vi "test_MultipleSessionsReserved_CallCreateSession_ReturnsErrorForTooManySessions.vi"(8 "error in":errorcluster) -> (0 "error out":errorcluster, 2 "result":string, 3 "pass":bool)   [LabVIEW 2020, in "MeasurementServerTests.lvlib"]
uses:
  MeasurementServerTests.lvlib
  3a947300-8ba6-4980-845e-9b7eeaceb0a3.vi
  Helpers/Fake Instrument/Fake Instrument.lvclass
  \\tsclient\C/dev/measurementlink-labview/Source/Runtime/MeasurementLink Instrument/IInstrument/IInstrument.lvclass
  Runtime/MeasurementLink Measurement Server/Helpers/Error Strings Global Internal.vi
  Runtime/MeasurementLink Session Management/Session Reservation/Create Sessions Impl.vi
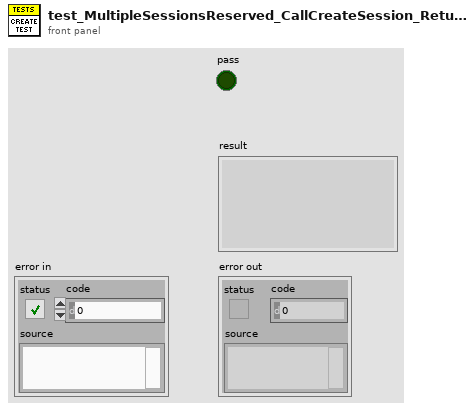
[diagram p1: front panel]
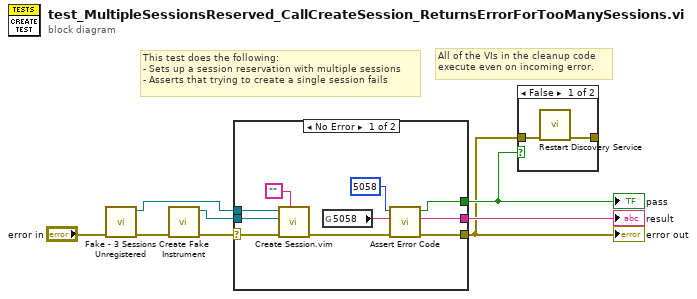
[diagram p0: block diagram]
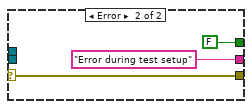
[diagram p2: hidden frame]
diagram:
  # "All of the VIs in the cleanup code\nexecute even on incoming error."
  # "This test does the following:\n- Sets up a session reservation with multiple sessions\n- Asserts that trying to create a single session fails"
  n1 = call "Fake - 3 Sessions Unregistered.vi"("error in"="error in") -> ("error out"=w2:errorcluster, "session reservation out"=w1:refnum<class "Session Reservation.lvclass">)  [unwired: 9 in]
  n2 = call "Create Fake Instrument.vi"("error in"=w2) -> ("error out"=w5:errorcluster, "fake instrument out"=w4:refnum<class "Fake Instrument.lvclass">)  [unwired: 9 in]
  n3 = case shown="No Error" w5 {
    selector: w5 -> [w16 w19]
    tunnel: [w10 w19] -> w6
    tunnel: [w14 FALSE] -> w7
    tunnel: [w9 "Error during test setup" ("f")] -> w8
    tunnel: w4 -> [w18 _]
    tunnel: w1 -> [w17 _]
    frame No Error {
      n4 = call "Create Session.vim"("session type"="", "error in"=w16, "instrument"=w18, "session reservation in"=w17) -> ("error out"=w15:errorcluster)  [unwired: 4 in, 3 out]
      n5 = global read "Error Strings Global Internal.vi" "5058"() -> (w11:string)
      n6 = call "Assert Error Code.vi"("error in"=w15, "expected error description"=w11, "expected error code"=5058) -> ("error out"=w10:errorcluster, "details"=w9:string, "error code match?"=w14:bool)  [unwired: 6 in]
    }
    frame Error {
    }
  }
  "error out" <- w6
  "pass" <- w7
  "result" <- w8
  n7 = case shown="False" w7 {
    tunnel: w6 -> [w23 _]
    tunnel: [w22 _] -> _
    frame False {
      n8 = call "Restart Discovery Service.vi"("error in"=w23) -> ("error out"=w22:errorcluster)  [unwired: 10 in]
    }
    frame True {
    }
  }
